vi "Parameters.vi"(8 "error in (no error)":errorcluster, 11 "Template Test Case In":refnum<class "Numeric Keypad Test.lvclass">) -> (0 "error out":errorcluster, 2 "Parameters":T1(array[cluster]))   [LabVIEW 2020, in "Numeric Keypad Test.lvclass"]
doc: "This VI defines the parameters used for execution. When LUnit runs the test case, it will run it once for every parameter in the array and collect the results.\n\nDuring test execution, the parameters are available in the class wire within the test VI."
uses:
  Numeric Keypad Test.lvclass
  C:/Program Files (x86)/National Instruments/LabVIEW 2020/vi.lib/Astemes/LUnit Parameterized/Parameterized Test Case/Parameterized Test Case.lvclass
  <vilib>/Astemes/LUnit Parameterized/Parameterized Test Case/Parameterized Test Case.lvclass
  Parameters.ctl
  Numeric Keypad Test.lvclass/Numeric Keypad Test.ctl
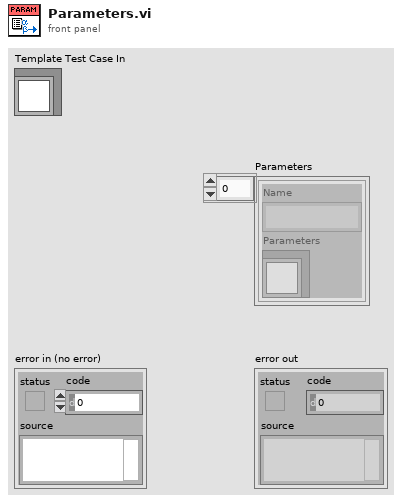
[diagram p1: front panel]
types:
  T1 = cluster{"Name":string, "Parameters":refnum<class "Parameterized Test Case.lvclass">}[]
  T2 = typedef "Numeric Keypad Test.lvclass/Parameters.ctl" = cluster{"Current":string, "Target":string, "Shortest":string}
  T3 = cluster{"Scenario":string, "Parameters":refnum<class "Numeric Keypad Test.lvclass">}[]
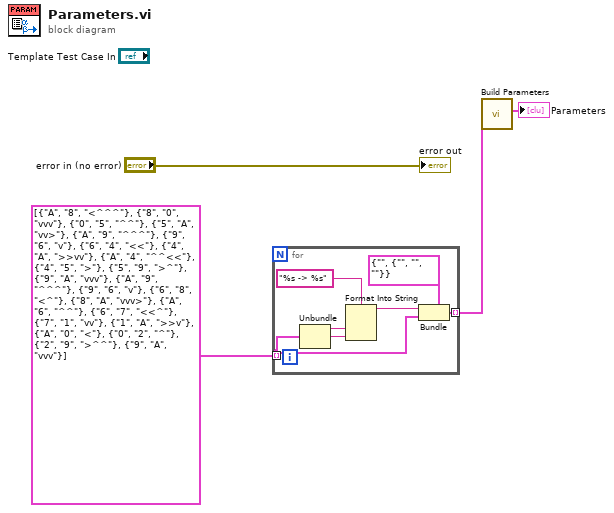
[diagram p0: block diagram]
diagram:
  n1 = for {
    tunnel: T2[] [{"Current"="A", "Target"="8", "Shortest"="<^^^"}, {"Current"="8", "Target"="0", "Shortest"="vvv"}, {"Current"="0", "Target"="5", "Shortest"="^^"}, {"Current"="5", "Target"="A", "Shortest"="vv>"}, {"Current"="A", "Target"="9", "Shortest"="^^^"}, {"Current"="9", "Target"="6", "Shortest"="v"}, {"Current"="6", "Target"="4", "Shortest"="<<"}, {"Current"="4", "Target"="A", "Shortest"=">>vv"}, {"Current"="A", "Target"="4", "Shortest"="^^<<"}, {"Current"="4", "Target"="5", "Shortest"=">"}, {"Current"="5", "Target"="9", "Shortest"=">^"}, {"Current"="9", "Target"="A", "Shortest"="vvv"}, {"Current"="A", "Target"="9", "Shortest"="^^^"}, {"Current"="9", "Target"="6", "Shortest"="v"}, {"Current"="6", "Target"="8", "Shortest"="<^"}, {"Current"="8", "Target"="A", "Shortest"="vvv>"}, {"Current"="A", "Target"="6", "Shortest"="^^"}, {"Current"="6", "Target"="7", "Shortest"="<<^"}, {"Current"="7", "Target"="1", "Shortest"="vv"}, {"Current"="1", "Target"="A", "Shortest"=">>v"}, {"Current"="A", "Target"="0", "Shortest"="<"}, {"Current"="0", "Target"="2", "Shortest"="^"}, {"Current"="2", "Target"="9", "Shortest"=">^^"}, {"Current"="9", "Target"="A", "Shortest"="vvv"}] -> [w6] mode=indexing
    tunnel: [w5] -> w1 mode=indexing
    n2 = Unbundle(w6) -> ("Current"=w8:string, "Target"=w7:string)  [unwired: 1 out]
    n3 = Format Into String(format string="%s -> %s", w8, w7) -> (resulting string=w9:string)  [unwired: 2 in, 1 out]
    n4 = Bundle(cluster=cluster{"Scenario":string, "Parameters":T2} {"Scenario"="", "Parameters"={"Current"="", "Target"="", "Shortest"=""}}, "Scenario"=w9, "Parameters"=w6) -> (w5:cluster{"Scenario":string, "Parameters":T2})
  }
  n5 = call "Build Parameters.vi"("Scenarios In"=w1) -> ("Scenarios out"=→"Parameters":T3)  [unwired: 10 in]
  "error out" <- "error in (no error)"
